vi "BMP085 Initialize.vi"(4 "Allow multiple opens?":bool=TRUE, 6 "I2C User Configuration":T1, 7 "Oversampling Setting (oss)":T3(ring), 8 "error in (no error)":errorcluster, 10 "Slave Address (7-bit)":u8=119 format="%.0x", 11 "Channel Name":tag="A/I2C") -> (0 "error out":errorcluster, 3 "BMP085 (GY-65) out":refnum<class "BMP085 (GY-65).lvclass">)   [LabVIEW 2015, in "BMP085 (RT).lvlib"]
uses:
  BMP085 (RT).lvlib
  BMP085 (GY-65).lvclass
  <vilib>/myRIO/Instrument Drivers/Onboard IO/I2C/typedefs/I2C User Configuration.ctl
  <vilib>/myRIO/Instrument Drivers/Onboard IO/I2C/typedefs/I2C Transfer Rate.ctl
  <vilib>/myRIO/Instrument Drivers/Onboard IO/I2C/I2C.lvlib
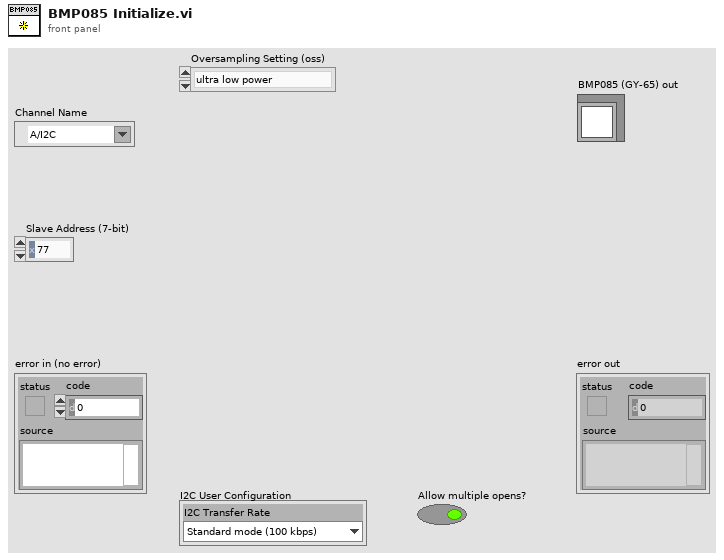
[diagram p1: front panel]
types:
  T1 = typedef "I2C.lvlib/I2C User Configuration.ctl" = cluster{"I2C Transfer Rate":T2}
  T2 = typedef "I2C.lvlib/I2C Transfer Rate.ctl" = enum16{"Standard mode (100 kbps)", "Fast mode (400 kbps)"}
  T3 = enum8{"ultra low power", "standard", "high resolution", "ultra high resolution"}
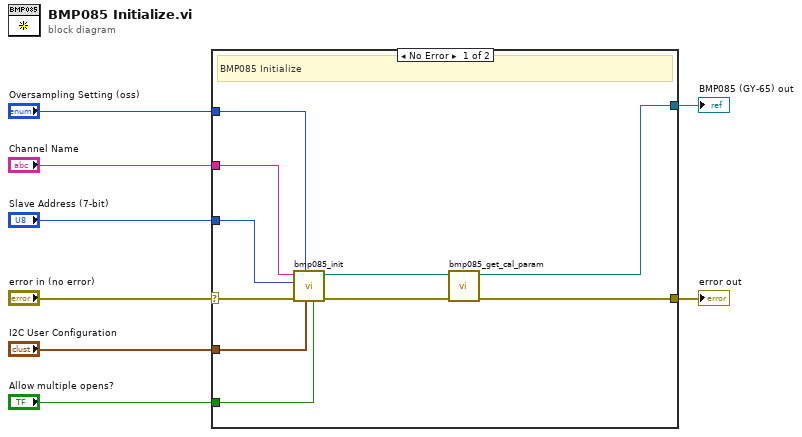
[diagram p0: block diagram]
diagram:
  n1 = case shown="No Error" "error in (no error)" {
    selector: "error in (no error)" -> [w17 w19]
    tunnel: [w16 w19] -> w7
    tunnel: [w14 _] -> w6
    tunnel: "Oversampling Setting (oss)" -> [w13 _]
    tunnel: "Channel Name" -> [w12 _]
    tunnel: "Slave Address (7-bit)" -> [w11 _]
    tunnel: "I2C User Configuration" -> [w10 _]
    tunnel: "Allow multiple opens?" -> [w9 _]
    frame No Error {
      # "BMP085 Initialize"
      n2 = call "bmp085_init.vi"("Allow multiple opens?"=w9, "I2C User Configuration"=w10, "Oversampling Setting (oss)"=w13, "error in (no error)"=w17, "Slave Address (7-bit)"=w11, "Channel Name"=w12) -> ("error out"=w18:errorcluster, "BMP085 (GY-65) out"=w15:refnum<class "BMP085 (GY-65).lvclass">)  [unwired: 4 in]
      n3 = call "bmp085_get_cal_param.vi"("error in (no error)"=w18, "BMP085 (GY-65) in"=w15) -> ("error out"=w16:errorcluster, "BMP085 (GY-65) out"=w14:refnum<class "BMP085 (GY-65).lvclass">)  [unwired: 8 in]
    }
    frame Error {
    }
  }
  "error out" <- w7
  "BMP085 (GY-65) out" <- w6
